vi "svfa_Generate Contiguous Bands from Bandwidth Profile.vi"(10 "frequency range [Hz]":cluster{"start":dbl, "stop":dbl}={"start"=0.0, "stop"=20000.0} {"stop" format="%.2f"; "start" format="%.2f"}, 11 "frequency resolution profile in":cluster{"f center":dbl, "bandwidth":dbl}[](array[cluster])=[{"f center"=0.0, "bandwidth"=6.25}, {"f center"=1600.0, "bandwidth"=6.25}, {"f center"=1600.0, "bandwidth"=12.5}, {"f center"=3200.0, "bandwidth"=12.5}, {"f center"=3200.0, "bandwidth"=25.0}, {"f center"=6400.0, "bandwidth"=25.0}, {"f center"=6400.0, "bandwidth"=50.0}, {"f center"=12800.0, "bandwidth"=50.0}, {"f center"=12800.0, "bandwidth"=100.0}, {"f center"=20000.0, "bandwidth"=100.0}]) -> (2 "band specifications [Hz]":T1(array[cluster]) {"bandwidth" format="%_6f"; "f center" format="%_6f"; "f high" format="%_6f"; "f low" format="%_6f"}, 3 "frequency resolution profile out":cluster{dbl, dbl}[](graph))   [LabVIEW 2017]
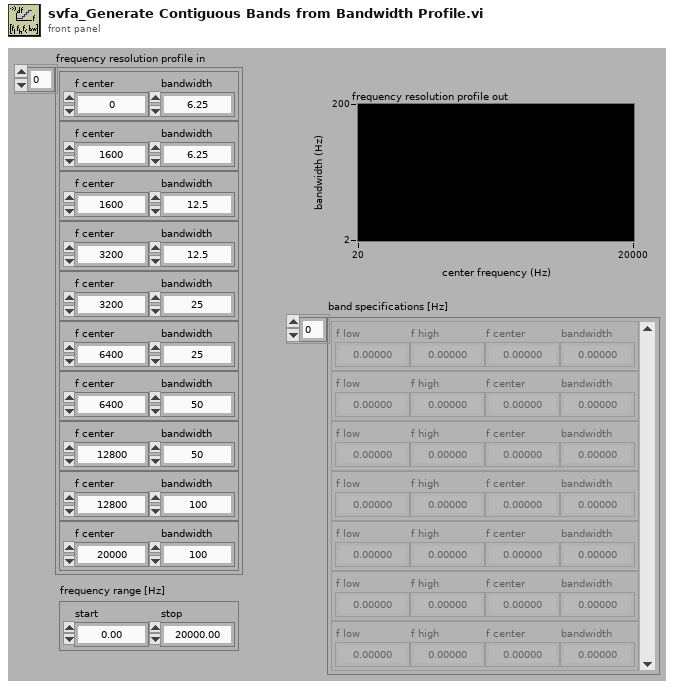
[diagram p1: front panel]
types:
  T1 = cluster{"f low":dbl, "f high":dbl, "f center":dbl, "bandwidth":dbl}[]
  T2 = cluster{"f low":dbl, "f high":dbl, "f center":dbl, "bandwidth":dbl}
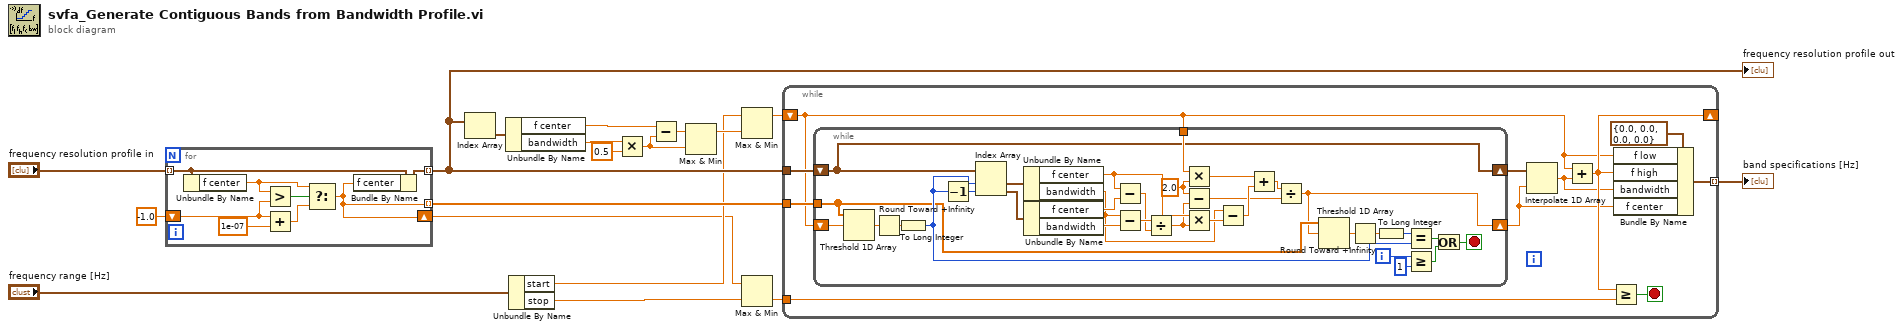
[diagram p0: block diagram]
diagram:
  n1 = for {
    tunnel: "frequency resolution profile in" -> [w21] mode=indexing
    shift-right: [w19] -> w1
    shift-left: -1.0 ("f0") -> [w26]
    tunnel: [w22] -> w8 mode=indexing
    tunnel: [w19] -> w7 mode=indexing
    n2 = Unbundle By Name(w21) -> ("f center"=w23:dbl)
    n3 = Greater?(x=w23, y=w26) -> (0:w25:bool)
    n4 = Add(x=w26, y=1e-07 ("f0")) -> (x+y=w24:dbl)
    n5 = Select(t=w23, s=w25, f=w24) -> (s? t:f=w19:dbl)
    n6 = Bundle By Name(cluster=w21, "f center"=w19) -> (w22:cluster{"f center":dbl, "bandwidth":dbl})
  }
  "frequency resolution profile out" <- w8
  n7 = Index Array(array=w8) -> (element=w10:cluster{"f center":dbl, "bandwidth":dbl})  [unwired: 1 in]
  n8 = Unbundle By Name(w10) -> ("f center"=w13:dbl, "bandwidth"=w11:dbl)
  n9 = Unbundle By Name("frequency range [Hz]") -> ("start"=w4:dbl, "stop"=w3:dbl)
  n10 = Multiply(x=w11, y=0.5) -> (x*y=w14:dbl)
  n11 = Subtract(x=w13, y=w14) -> (x-y=w15:dbl)
  n12 = Max & Min(x=w15, y=w14) -> (max(x,y)=w16:dbl)  [unwired: 1 out]
  n13 = Max & Min(x=w4, y=w16) -> (max(x,y)=w9:dbl)  [unwired: 1 out]
  n14 = Max & Min(x=w1, y=w3) -> (min(x,y)=w2:dbl)  [unwired: 1 out]
  n15 = while {
    tunnel: w8 -> [w37]
    tunnel: w7 -> [w31]
    shift-right: [w33] -> _
    shift-left: w9 -> [w30]
    tunnel: w2 -> [w35]
    tunnel: [w34] -> w6 mode=indexing
    stop <- w36 stop-if-true
    n16 = while {
      tunnel: w30 -> [w54]
      shift-right: [w53] -> w32
      shift-left: w37 -> [w53]
      tunnel: w31 -> [w39]
      shift-right: [w38] -> w29
      shift-left: w30 -> [w50]
      i -> [w45]
      stop <- w41 stop-if-true
      w60 = 2.0 ("x")
      n17 = Threshold 1D Array(2:w50, 3:w39) -> (0:w51:dbl)  [unwired: 1 in]
      n18 = Round Toward +Infinity(x=w51) -> (ceil(x): smallest int >= x=w52:dbl)
      n19 = To Long Integer(number=w52) -> (32bit integer=w40:i32)
      n20 = Decrement(x=w40) -> (x-1=w55:i32)
      n21 = Index Array(array=w53, index #1=w40, index #2=w55) -> (element #1=w69:cluster{"f center":dbl, "bandwidth":dbl}, element #2=w68:cluster{"f center":dbl, "bandwidth":dbl})
      n22 = Unbundle By Name(w69) -> ("f center"=w62:dbl, "bandwidth"=w46:dbl)
      n23 = Unbundle By Name(w68) -> ("f center"=w65:dbl, "bandwidth"=w64:dbl)
      n24 = Subtract(x=w62, y=w65) -> (x-y=w66:dbl)
      n25 = Subtract(x=w46, y=w64) -> (x-y=w67:dbl)
      n26 = Divide(x=w67, y=w66) -> (x/y=w61:dbl)
      n27 = Multiply(x=w54, y=w60) -> (x*y=w59:dbl)
      n28 = Subtract(x=w60, y=w61) -> (x-y=w56:dbl)
      n29 = Multiply(x=w62, y=w61) -> (x*y=w63:dbl)
      n30 = Subtract(x=w46, y=w63) -> (x-y=w58:dbl)
      n31 = Add(x=w59, y=w58) -> (x+y=w57:dbl)
      n32 = Divide(x=w57, y=w56) -> (x/y=w38:dbl)
      n33 = Threshold 1D Array(2:w38, 3:w39) -> (0:w48:dbl)  [unwired: 1 in]
      n34 = Round Toward +Infinity(x=w48) -> (ceil(x): smallest int >= x=w49:dbl)
      n35 = To Long Integer(number=w49) -> (32bit integer=w47:i32)
      n36 = Equal?(x=w47, y=w40) -> (x = y?=w42:bool)
      n37 = Greater Or Equal?(x=w45, y=1) -> (x >= y?=w43:bool)
      n38 = Or(x=w42, y=w43) -> (x .or. y?=w41:bool)
    }
    n39 = Interpolate 1D Array(1:w29, 2:w32) -> (0:w28:dbl)
    n40 = Add(x=w30, y=w28) -> (x+y=w33:dbl)
    n41 = Greater Or Equal?(x=w33, y=w35) -> (x >= y?=w36:bool)
    n42 = Bundle By Name(cluster=T2 {"f low"=0.0, "f high"=0.0, "f center"=0.0, "bandwidth"=0.0} ("Bandedge frequencies [Hz]"), "f low"=w30, "f high"=w33, "bandwidth"=w28, "f center"=w29) -> (w34:T2)
  }
  "band specifications [Hz]" <- w6
